vi "MeasureRMS.vi"(2 "rate":dbl=1000.0, 3 "number of samples":i32=100) -> (0 "data":dynamicdata(graph), 1 "AC estimate (Vrms)":dbl format="%0.2f")   [LabVIEW 2015]
uses:
  <vilib>/Analysis/NI_AALPro.lvlib
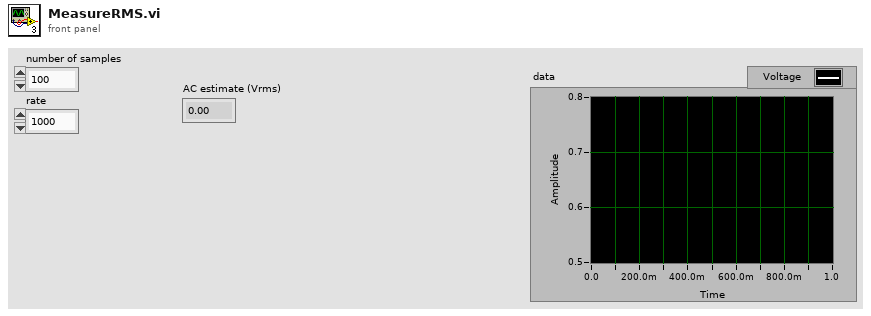
[diagram p1: front panel]
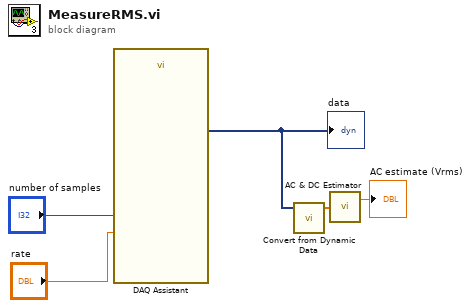
[diagram p0: block diagram]
diagram:
  n1 = call "DAQ Assistant"("rate"="rate", "number of samples"="number of samples") -> ("data"=w3:dynamicdata)  [unwired: 15 in, 2 out]
  "data" <- w3
  n2 = call "Convert from Dynamic Data"("Dynamic Data Type"=w3) -> ("Array"=w2:dbl[])  [unwired: 3 in]
  n3 = call <vilib>:"AC & DC Estimator.vi"("Signal (V)"=w2) -> ("AC estimate (Vrms)"=→"AC estimate (Vrms)":dbl)  [unwired: 1 out]
